vi "Dashboard Main.vi"() -> ()   [LabVIEW 2018]
uses:
  <vilib>/Rock Robotics/WPI/Camera/WPI_CameraExposure Values.ctl
  <vilib>/Rock Robotics/WPI/Camera/WPI_CameraWhite Balance Values.ctl
  <vilib>/Rock Robotics/WPI/Camera/WPI_CameraSettings Read MJPG.ctl
  <vilib>/Rock Robotics/WPI/Camera/WPI_CameraImageSize.ctl
  <vilib>/Utility/miscctls.llb/LVRowAndColumnTypeDef.ctl
  <vilib>/event_ctls.llb/eventvkey.ctl
  <vilib>/Rock Robotics/Network Tables/NT Read Numeric Array.vi
  <vilib>/Rock Robotics/WPI/Dashboard/WPI_DashboardLogging Global.vi
  <vilib>/Rock Robotics/Network Tables/NT Write Boolean.vi
  Vision Things/Dashboard globals.vi
  <vilib>/Utility/inputDevices.llb/keyboardAcquire.vi
  <vilib>/vision/NI_Vision_Development_Module.lvlib
  <vilib>/Rock Robotics/Network Tables/NT Write Variant.vi
panel:
  in  "Camera Settings Right":T1={"Frame Rate"=30, "Compression"=30, "Size"=1, "DB Camera Config"=FALSE} {"Frame Rate" scale=1.0..30.0; "Compression" scale=100.0..-1.0; "Size" items=["640x480", "320x240", "160x120"]}
  in  "Camera Name Right":string(combo)="No Camera Selection"
  out "Camera Perf":string
  in  "Camera Settings":T1={"Frame Rate"=30, "Compression"=30, "Size"=1, "DB Camera Config"=FALSE} {"Frame Rate" scale=1.0..30.0; "Compression" scale=100.0..-1.0; "Size" items=["640x480", "320x240", "160x120"]}
  in  "TCP":refnum<k5>
  in  "Rec Mode":enum32{"Stop", "Record", "Playback"}(radio)
  out "Robot IP":string
  out "Image Message":string="Timeout in Camera Communications"
  in  "Dashboard Tab":T2(tab)
  in  "Desired Target":T3(radio)
  in  "Select Auto":string(combo)="Select Autonomous ..."
  out "NT Connection":bool
  out "MotorChart R":cluster{"Numeric":dbl, "Numeric":dbl}(graph)
  out "MotorChart L":cluster{"Numeric":dbl, "Numeric":dbl}(graph)
  out "MotorSliders R":cluster{"MotorSlide1":dbl, "MotorSlide2":dbl} {"MotorSlide2" scale=-1.0..1.0 scale format="%#_2e"; "MotorSlide1" scale=-1.0..1.0 scale format="%#_2e"}
  out "MotorSliders L":cluster{"MotorSlide1":dbl, "MotorSlide2":dbl} {"MotorSlide2" scale=-1.0..1.0 scale format="%#_2e"; "MotorSlide1" scale=-1.0..1.0 scale format="%#_2e"}
  out "Gyro":dbl(knob) scale=0.0..360.0
  out "JS1 Z":dbl(slide) scale=-1.0..1.0 scale format="%#_2e"
  out "JS1 Graph":cluster{"X":dbl, "Y":dbl}[](graph)
  out "JS1 Buttons":T4
  out "JS2 Z":dbl(slide) scale=-1.0..1.0 scale format="%#_2e"
  out "JS2 Graph":cluster{"X":dbl, "Y":dbl}[](graph)
  out "JS2 Buttons":T4
  out "Mode":T5(ring)=enum."Auto Disabled"
  out "Right Camera Perf":cluster{"Bandwidth (Mbps)":dbl, "FPS":dbl}
  in  "Auton Side":enum16{"Front", "Left", "Right"}(ring)
  in  "Side Code":enum16{"Right", "Left"}(ring)
  in  "Slot #":enum16{"3", "2", "1"}(ring)
  out "Auton String":string
  in  "Starting Postion":enum16{"2R", "2L", "1L", "1R", "1M"}(ring)
  out "Camera Image Right":T6(plugin-control)
  in  "DB/String 9":string
  in  "DB/String 8":string
  in  "DB/String 7":string
  in  "DB/String 6":string
  in  "DB/String 5":string
  in  "DB/String 4":string
  in  "DB/String 3":string
  in  "DB/String 2":string
  in  "DB/String 1":string
  in  "DB/String 0":string
  in  "DB/Slider 0":dbl(slide) scale=0.0..5.0
  in  "DB/Slider 1":dbl(slide) scale=0.0..5.0
  in  "DB/Slider 2":dbl(slide) scale=0.0..5.0
  in  "DB/Slider 3":dbl(slide) scale=0.0..5.0
  out "DB/LED 3":bool
  out "DB/LED 2":bool
  out "DB/LED 1":bool
  out "DB/LED 0":bool
  in  "DB/Button 3":bool
  in  "DB/Button 2":bool
  in  "DB/Button 1":bool
  in  "DB/Button 0":bool caption="New Name"
  in  "Test Slider":dbl(slide) scale=0.0..100.0 scale format="%#_3g"
  in  "On/Off":bool caption="Solenoid"
  in  "Test Name":u16(ring) items=["Select the test to run..."]
  in  "Test Tree":string(tree)
  in  "Motor":cluster{"Value":dbl, "Enable":bool} {"Value" scale=-1.0..1.0 scale format="%#_3g"}
  out "Progress":T7 {"Test Progress" scale=0.0..100.0}
  in  "Rev/Fwd":cluster{"Forward":bool, "Reverse":bool}
  in  "Test Ring":u16(ring) items=["Monochrome", "Color"]
  out "Cmd Status":string
  in  "Execute Command":bool
  in  "Command Params":string[][](table)
  in  "Command Selection":i32(listbox)
  in  "CheckList":i32(listbox)
  out "Tree":string(tree)
  out "Camera Image":T6(plugin-control)
  out "Background":bool
  in  "Camera Name":string(combo)="No Camera Selection"
  # "HW"
  # "HW"
  # "Joysticks"
  # "Drive Motors"
  # "Front"
  # "Right"
  # "Left"
  # "Back"
  # "This tab is a great place for autonomous settings and robot-specific values.\nPlace controls and indicators inside this tab and match name to\nDashboard Variables on robot. You can also delete this comment."
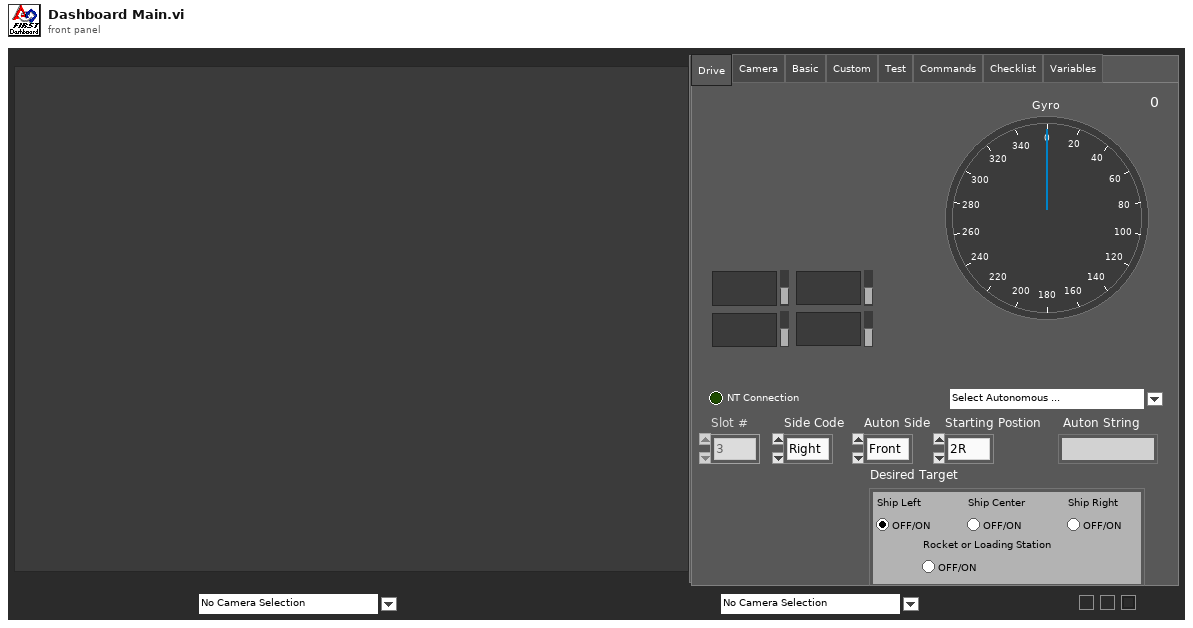
[diagram p1: front panel]
types:
  T1 = cluster{"Frame Rate":i32, "Compression":i32, "Size":u16, "DB Camera Config":bool}
  T2 = enum32{"Drive", "Camera", "Basic", "Custom", "Test", "Commands", "Checklist", "Variables"}
  T3 = enum32{"Ship Left", "Ship Center", "Ship Right", "Rocket or Loading Station"}
  T4 = cluster{bool, bool, bool, bool, bool, bool, bool, bool, bool, bool, bool, bool}
  T5 = enum8{"Tele-Op Disabled", "Tele-Op Enabled", "Auto Disabled", "Auto Enabled", "Test Disabled", "Test Enabled", "Disconnected", "No Code", "E-Stop"}
  T6 = typedef "IMAQ Image.ctl" = refnum<image>
  T7 = cluster{"Test Progress":u8, "Test Progress Text":string}
  T8 = cluster{"Save Path":path, "Interval (s)":dbl, "Keep":i32}
  T9 = typedef "Image Type" = u32
  T10 = cluster{"IDs":cluster{"RPC field ID":u16, "Unique ID":u16}, "String":string}
  T11 = enum8{"Enabled", "Disabled", "Disabled and Grayed Out"}
  T12 = enum16{"0", "1", "2", "3", "4", "5", "6", "7", "8", "9", "A", "B", "C", "D", "E", "F", "G", "H", "I", "J", "K", "L", "M", "N", "O", "P", "Q", "R", "S", "T", "U", "V", "W", "X", "Y", "Z", "F1", "F2", "F3", "F4", "F5", "F6", "F7", "F8", "F9", "F10", "F11", "F12", "F13", "F14", "F15", "ADD", "BACK", "BACKSLASH", "CAPITAL", "COMMA", "DECIMAL", "DELETE", "DIVIDE", "DOWN", "END", "EQUALS", "ESCAPE", "GRAVE (`)", "HOME", "INSERT", "LBRACKET", "LCONTROL", "LEFT", "L ALT", "LSHIFT", "LWIN", "MINUS", "MULTIPLY", "NEXT", "NUMLOCK", "NUMPAD_0", "NUMPAD_1", "NUMPAD_2", "NUMPAD_3", "NUMPAD_4", "NUMPAD_5", "NUMPAD_6", "NUMPAD_7", "NUMPAD_8", "NUMPAD_9", "PAUSE", "PERIOD", "PRIOR (PG UP)", "RBRACKET", "RCONTROL", "RETURN", "RIGHT", "R ALT", "RSHIFT", "RWIN", "SCROLL", "SEMICOLON", "SLASH", "SPACE", "SUBTRACT", "TAB", "UP", "ENTER (num pad)", "' (quote)"}[]
  T13 = enum16{"0", "1", "2", "3", "4", "5", "6", "7", "8", "9", "A", "B", "C", "D", "E", "F", "G", "H", "I", "J", "K", "L", "M", "N", "O", "P", "Q", "R", "S", "T", "U", "V", "W", "X", "Y", "Z", "F1", "F2", "F3", "F4", "F5", "F6", "F7", "F8", "F9", "F10", "F11", "F12", "F13", "F14", "F15", "ADD", "BACK", "BACKSLASH", "CAPITAL", "COMMA", "DECIMAL", "DELETE", "DIVIDE", "DOWN", "END", "EQUALS", "ESCAPE", "GRAVE (`)", "HOME", "INSERT", "LBRACKET", "LCONTROL", "LEFT", "L ALT", "LSHIFT", "LWIN", "MINUS", "MULTIPLY", "NEXT", "NUMLOCK", "NUMPAD_0", "NUMPAD_1", "NUMPAD_2", "NUMPAD_3", "NUMPAD_4", "NUMPAD_5", "NUMPAD_6", "NUMPAD_7", "NUMPAD_8", "NUMPAD_9", "PAUSE", "PERIOD", "PRIOR (PG UP)", "RBRACKET", "RCONTROL", "RETURN", "RIGHT", "R ALT", "RSHIFT", "RWIN", "SCROLL", "SEMICOLON", "SLASH", "SPACE", "SUBTRACT", "TAB", "UP", "ENTER (num pad)", "' (quote)"}
  T14 = typedef "WPI_CameraExposure Values.ctl" = enum16{"Auto", "Flicker-free 50 Hz", "Flicker-free 60 Hz", "Hold current", "Custom"}
  T15 = typedef "WPI_CameraWhite Balance Values.ctl" = enum16{"Auto", "Fixed indoor", "Fixed outdoor 1", "Fixed outdoor 2", "Fixed fluorescent 1", "Fixed fluorescent 2", "Hold current", "Custom"}
  T16 = cluster{"Exposure":T14, "Exposure (%)":dbl, "Brightness":i32, "White Balance":T15, "Color Temp (K)":dbl}
  T17 = typedef "WPI_CameraSettings Read MJPG.ctl" = cluster{"fps":i32, "compression":i32, "Image Size":T18, "Config Shown":bool}
  T18 = typedef "WPI_CameraImageSize.ctl" = enum16{"640x480", "320x240", "160x120", "Custom"}
  T19 = cluster{"Global Rectangle":i32[], "Contours":cluster{"Contour Type":u32, "ROI Type":u32, "Points":i32[]}[]}
  T20 = cluster{"Camera Name":string, string, "Saved DB Images Info":cluster{"Save Path":path, "Interval (s)":dbl, "Keep":i32}}
  T21 = cluster{"Corners":cluster{"X":sgl, "Y":sgl}[], "Orientation (degrees)":dbl, "Width":dbl, "Height":dbl, "Score":dbl}[]
  T22 = cluster{"Camera Name Right":string, string, "Saved DB Images Info":cluster{"Save Path":path, "Interval (s)":dbl, "Keep":i32}}
  T23 = cluster{"Camera Image":refnum<vi>, "Dashboard Tab":refnum<vi>, "Background":refnum<vi>, "Rec Mode":refnum<vi>, "Test Slider":refnum<vi>, "On/Off ":refnum<vi>, "Test Ring":refnum<vi>, "Rev/Fwd":refnum<vi>, "Test Name":refnum<vi>, "Motor":refnum<vi>, "Progress":refnum<vi>, "CheckList":refnum<vi>, "Tree":refnum<vi>, "Test Tree":refnum<vi>, "Command Params":refnum<vi>, "Command Selection":refnum<vi>, "Execute Command":refnum<vi>, "Cmd Status":refnum<vi>, "Camera Settings":refnum<vi>, "Camera Name":refnum<vi>, "Camera Perf":refnum<vi>, "Camera Settings Right":refnum<vi>, "Camera Name Right":refnum<vi>, "Camera Image Right":refnum<vi>}
  T24 = cluster{"Error Strings":string, "Disable Counts":cluster{u16, u16}, "Rail Faults":cluster{u16, u16, u16}, "Robot IP":string, "DB Mode":u8, "Event Info":cluster{"Name":string, "Type":u8, "Number":u16, "Replay":u8}}
  T25 = cluster{"Storage":cluster{"Disk Free":u64, "RAM Block":u32, "RAM free":u32}, "CPU Utilization":cluster{"CPU % ISR":sgl, "CPU % Time Crit":sgl, "CPU % Timed Str":sgl, "CPU % High":sgl, "CPU % Above":sgl, "CPU % Normal":sgl, "CPU % Low":sgl}, "CAN":cluster{"% Bus Utilization":sgl, "Bus Off Cnt":u32, "TX_FIFO Full Cnt":u32, "Receive Error Cnt":u8, "Transmit Error Cnt":u8}, "HID":cluster{"HID Outputs":u32, "Rumble Low":u16, "Rumble High":u16}[]}
  T26 = cluster{"Status bits":cluster{"Test Mode":bool, "Autonomous":bool, "Enabled":bool, "Code Start":bool, "Brownout":bool, "Reserved 2":bool, "Reserved 3":bool, "E-Stop":bool}, "Code Trace":cluster{"Disabled":bool, "TeleOp":bool, "Auto":bool, "Test":bool}, "Controller Type":enum16{"unknown", "cRIO", "roboRio"}, "Code?":enum16{"unknown", "noCode", "code"}, "Battery V":dbl}
  T27 = cluster{"Control Bits":cluster{"TestMode":bool, "Autonomous":bool, "Enabled":bool, "FMS Present":bool, bool, bool, bool, "E-Stop":bool}, "Team Station ":u8, "Countdown":sgl, "Joystick Values":cluster{"Axes":dbl[], "Buttons":bool[], "POVs":i16[]}[]}
  T28 = cluster{"Axes":dbl[], "Buttons":bool[], "POVs":i16[]}[]
  T29 = cluster{"Increase in Left":dbl, "Increase in Right":dbl}[]
  T30 = cluster{"Axes":dbl[], "Buttons":bool[], "POVs":i16[]}
  T31 = cluster{"Buttons[0]":bool, "Buttons[1]":bool, "Buttons[2]":bool, "Buttons[3]":bool, "Buttons[4]":bool, "Buttons[5]":bool, "Buttons[6]":bool, "Buttons[7]":bool, "Buttons[8]":bool, "Buttons[9]":bool, "Buttons[10]":bool, "Buttons[11]":bool}
  T32 = cluster{"Operation":enum16{"Update", "Clear"}, "Color Box":u32}[]
  T33 = typedef "eventvkey.ctl" = enum16{"ASCII", "Enter", "Return", "Shift", "Ctrl", "Alt", "Cmd", "Opt", "Caps", "NumLock", "Clear", "Break", "Up", "Down", "Left", "Right", "Insert", "Delete", "Home", "End", "PageUp", "PageDown", "Escape", "Help", "Pause", "ScrollLock", "F1", "F2", "F3", "F4", "F5", "F6", "F7", "F8", "F9", "F10", "F11", "F12", "F13", "F14", "F15", "F16", "F17", "F18", "F19", "F20", "F21", "F22", "F23", "F24", "Play", "VolumeUp", "VolumeDown", "Mute", "Two Byte Char"}
  T34 = cluster{"Image Size":bool, "Image Type":bool, "Pixel Value":bool, "ROI Information":bool, "Zoom Factor":bool}
  T35 = cluster{"Operation":enum16{"Update", "Clear"}, "Color Box":u32}
  T36 = typedef "LVRowAndColumnTypeDef.ctl" = cluster{"Row":i32, "Column":i32}
  T37 = cluster{"Shift":bool, "Ctrl":bool, "Alt":bool, "Cmd":bool, "Opt":bool}
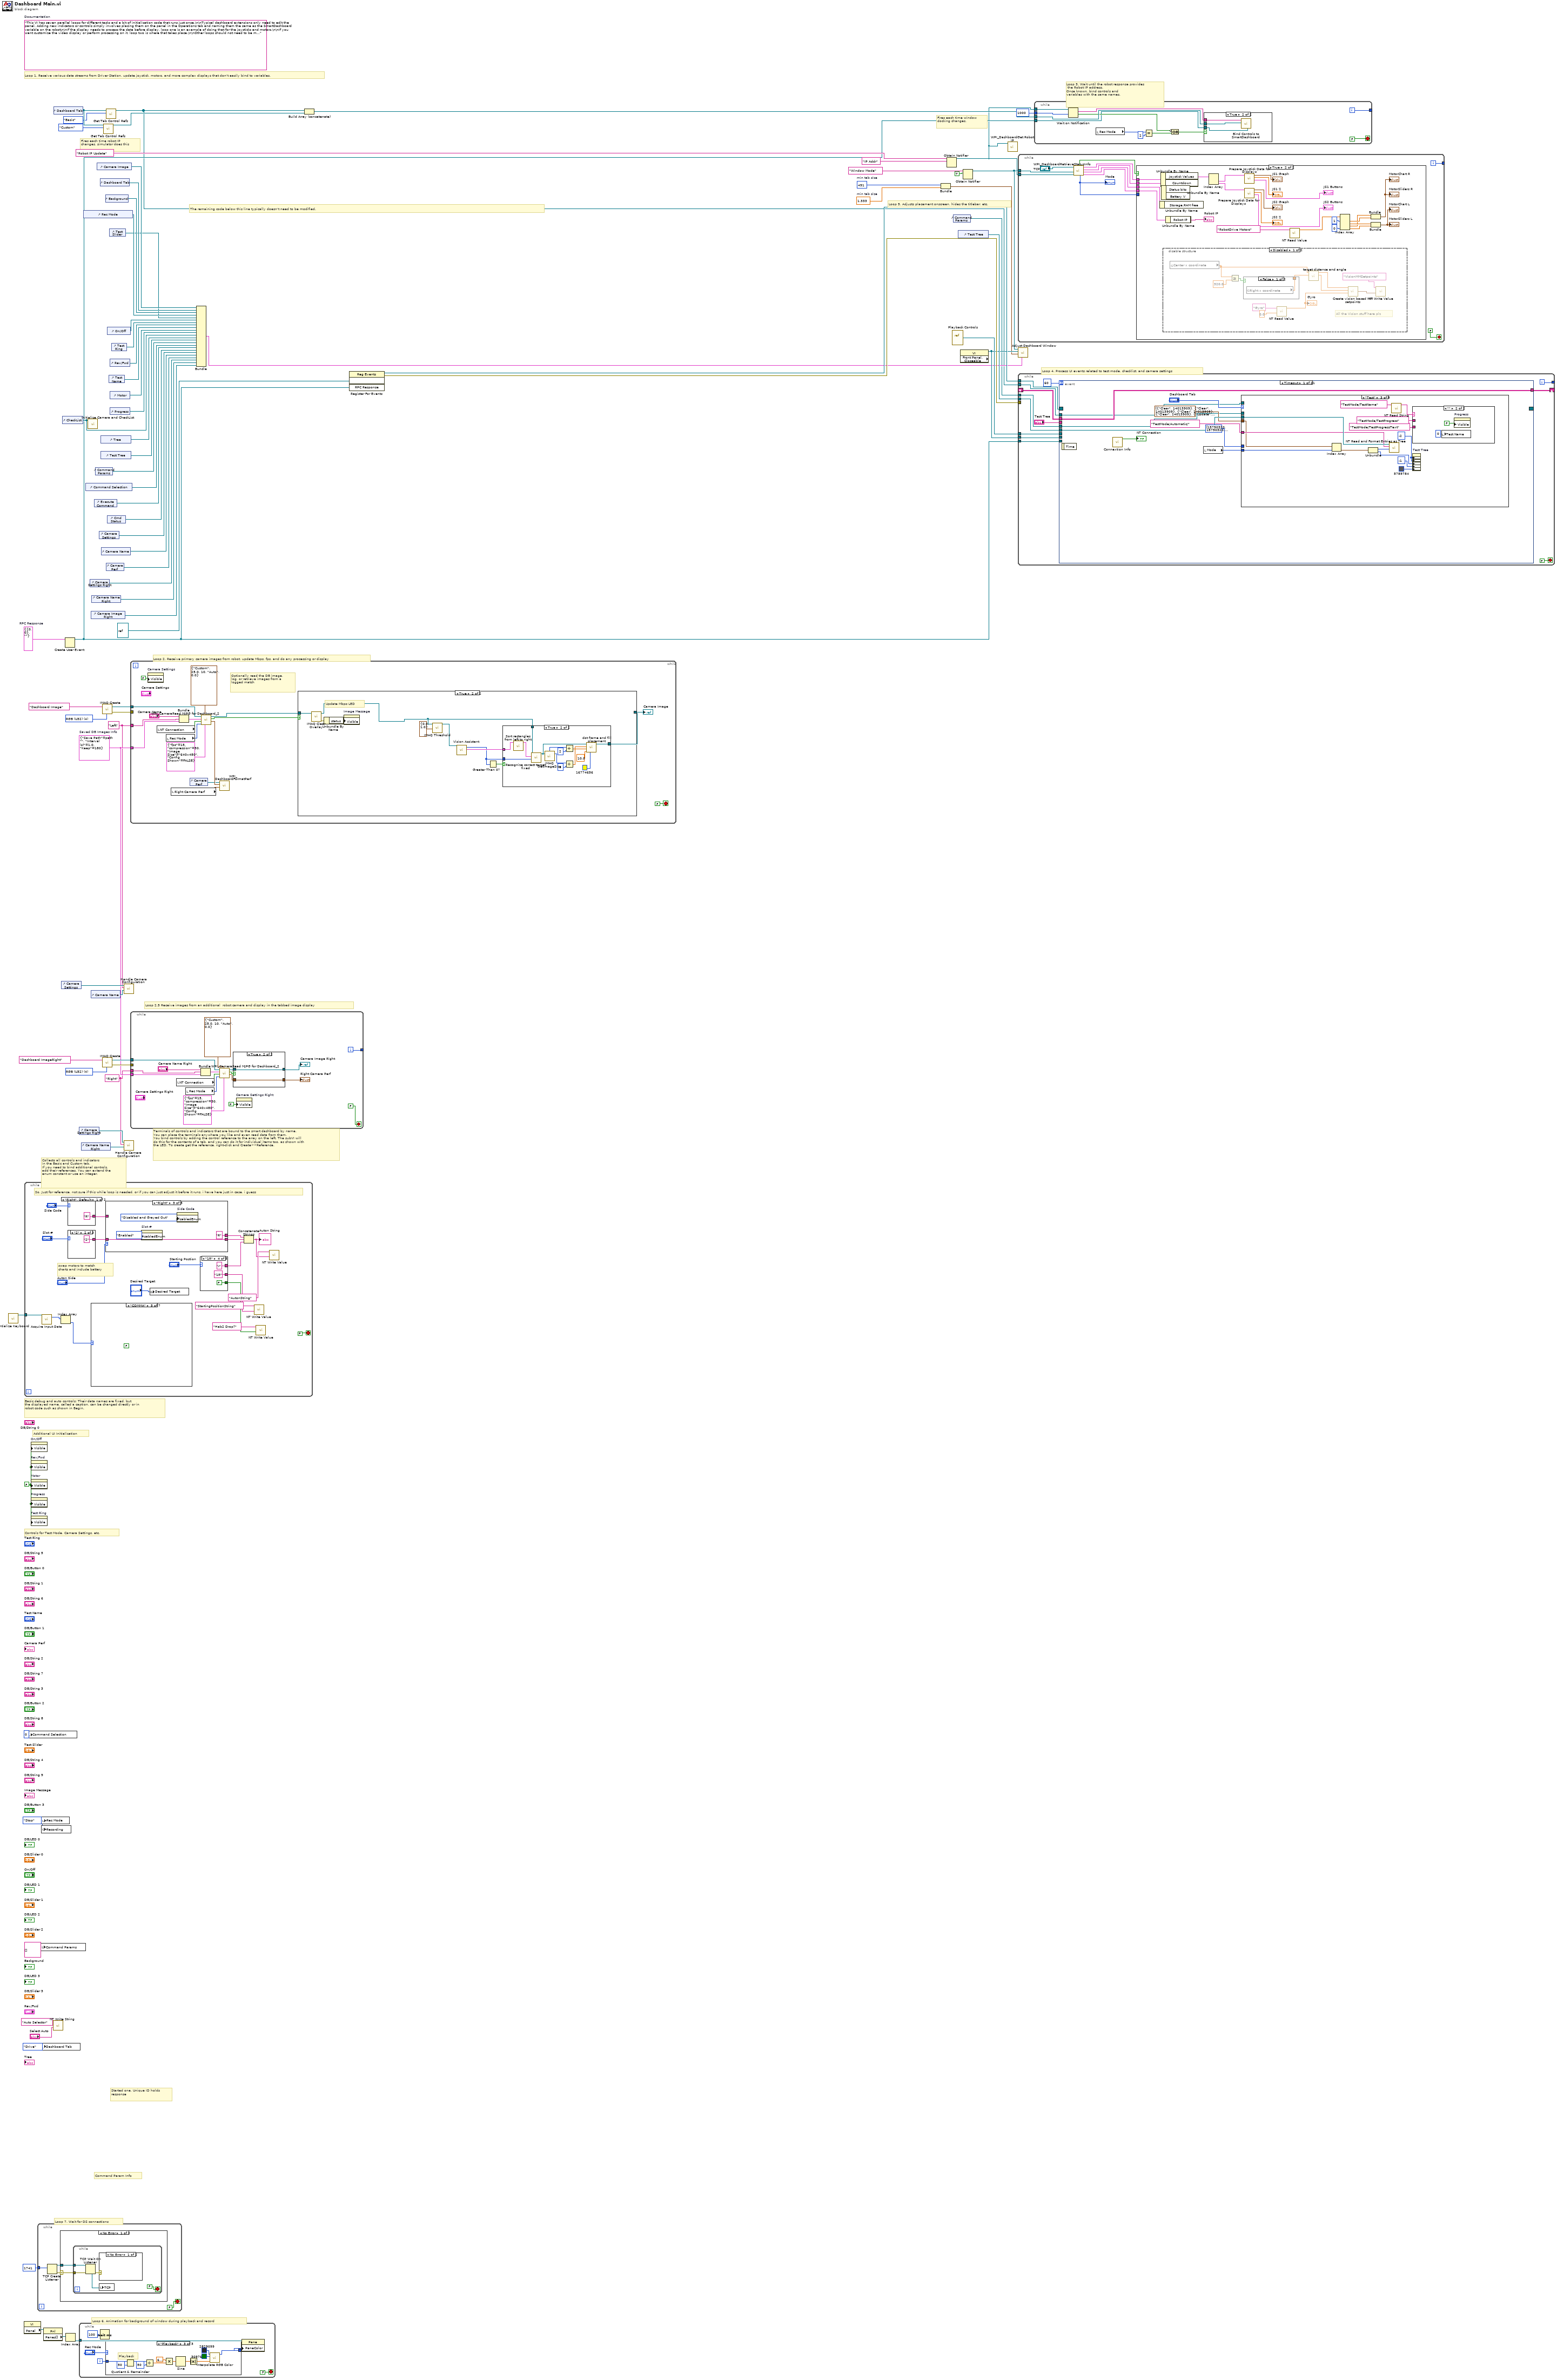
[diagram p0: block diagram]
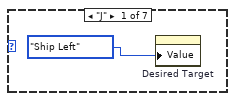
[diagram p2: hidden frame]
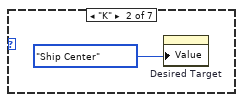
[diagram p3: hidden frame]
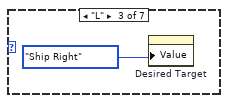
[diagram p4: hidden frame]
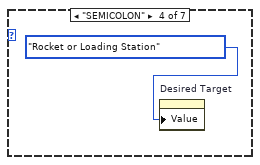
[diagram p5: hidden frame]
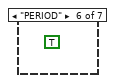
[diagram p6: hidden frame]
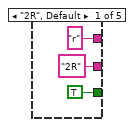
[diagram p8: hidden frame]
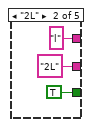
[diagram p9: hidden frame]
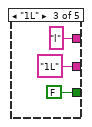
[diagram p10: hidden frame]
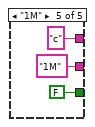
[diagram p11: hidden frame]
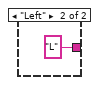
[diagram p12: hidden frame]
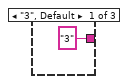
[diagram p13: hidden frame]
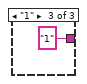
[diagram p14: hidden frame]
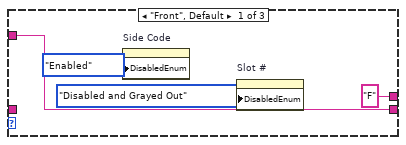
[diagram p15: hidden frame]
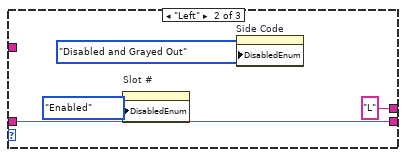
[diagram p16: hidden frame]
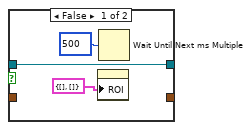
[diagram p17: hidden frame]
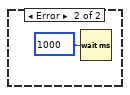
[diagram p18: hidden frame]
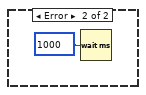
[diagram p19: hidden frame]
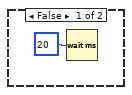
[diagram p20: hidden frame]
diagram:
  w5 = T8 {"Save Path"=path "", "Interval (s)"=1.0, "Keep"=180}  # Saved DB Images Info
  w4 = "Right"
  w3 = "Left"
  w15 = T9 4 items=["Grayscale (U8)", "Grayscale (I16)", "Grayscale (SGL)", "Complex (CSG)", "RGB (U32)", "HSL (U32)", "RGB (U64)"] ("Image Type")
  w31 = T10 {"IDs"={"RPC field ID"=0, "Unique ID"=0}, "String"=""}  # RPC Response
  w53 = 491  # min tab size
  w52 = 1.333  # min tab size
  w60 = enum32{"Stop", "Record", "Playback"}."Stop" ("Rec Mode")
  w37 = FALSE ("Visible")
  (unwired) "This VI has seven parallel loops for different tasks and a bit of initialization code that runs just once.\n\nTypical dashboard extensions only need to edit the panel. Adding new indicators or controls simply involves placing them on the panel in the Operations tab and naming them the same as the SmartDashboard variable on the robot\n\nIf the display needs to process the data before display, loop one is an example of doing that for the joysticks and motors.\n\nIf you want customize the video display or perform processing on it, loop two is where that takes place.\n\nOther loops should not need to be modified. They are pretty standard, and document the task they perform."  # Documentation
  w77 = T9 4 items=["Grayscale (U8)", "Grayscale (I16)", "Grayscale (SGL)", "Complex (CSG)", "RGB (U32)", "HSL (U32)", "RGB (U64)"] ("Image Type")
  # "Collects all controls and indicators\nin the Basic and Custom tab.\nIf you need to bind additional controls,\nadd their references. You can extend the\nenum constant or use an integer."
  # "Terminals of controls and indicators that are bound to the smart dashboard by name.\nYou can place the terminals anywhere you like and even read data from them.\nYou bind controls by adding the control reference to the array on the left. The subVI will\ndo this for the contents of a tab, and you can do it for individual items too, as shown with\nthe LED. To create get the reference, right-click and Create>>Reference."
  # "Loop 2.5 Receive images from an additional  robot camera and display in the tabbed image display"
  # "Command Param Info"
  # "Started one, Unique ID holds\nresponse"
  # "Loop 7. Wait for DS connections"
  # "Basic debug and auto controls: Their data names are fixed, but\nthe displayed name, called a caption, can be changed directly or in\nrobot code such as shown in Begin."
  # "Controls for Test Mode, Camera Settings, etc."
  # "Additional UI Initialization"
  # "Loop 6. Animation for background of window during playback and record"
  # "Fires each time robot IP\nchanges, simulator does this"
  # "Fires each time window\ndocking changes."
  # "The remaining code below this line typically doesn't need to be modified."
  # "Loop 4. Process UI events related to test mode, checklist, and camera settings"
  # "Loop 3. Wait until the robot response provides\n the Robot IP address.\nOnce known, bind controls and\nvariables with the same names."
  # "Loop 5. Adjusts placement onscreen, hides the titlebar, etc."
  # "Loop 1. Receive various data streams from Driver Station, update joystick, motors, and more complex displays that don't easily bind to variables."
  # "Loop 2. Receive primary camera images from robot, update Mbps, fps, and do any processing or display"
  n1 = call <vilib>:"Intialize Keyboard.vi"() -> ("device ID"=w2:refnum<k1>)  [unwired: 10 in, 1 out]
  n2 = property class="VI"() -> ("Panel"=w67:refnum<vi>)  [unwired: 2 in, 2 out]
  n3 = while {
    tunnel: w2 -> [w81]
    stop <- FALSE stop-if-true
    # "So, Just for reference, not sure if this while loop is needed, or if you can just adjust it before it runs, i have here just in case, i guess"
    # "swap motors to match\ncharts and include battery"
    n4 = call-poly <vilib>:"Acquire Input Data.vi"("device ID"=w81) -> ("keys pressed"=w80:T12)  [unwired: 16 in, 2 out]
    n5 = Index Array(array=w80) -> (element=w79:T13)  [unwired: 1 in]
    n6 = case shown="\"Right\", Default" "Side Code" {
      tunnel: ["R" "L"] -> w93
      frame "Right", Default {
      }
      frame "Left" {
      }
    }
    n7 = case shown="\"2\"" "Slot #" {
      tunnel: ["3" "2" "1"] -> w94
      frame "3", Default {
      }
      frame "2" {
      }
      frame "1" {
      }
    }
    n8 = case shown="\"COMMA\"" w79 {
      frame "J" {
        n9 = property on="Desired Target" class="RadioBtnsControl (strict)"("Value"=T3."Ship Left" ("Desired Target")) -> ()  [unwired: 2 in, 2 out]
      }
      frame "K" {
        n10 = property on="Desired Target" class="RadioBtnsControl (strict)"("Value"=T3."Ship Center" ("Desired Target")) -> ()  [unwired: 2 in, 2 out]
      }
      frame "L" {
        n11 = property on="Desired Target" class="RadioBtnsControl (strict)"("Value"=T3."Ship Right" ("Desired Target")) -> ()  [unwired: 2 in, 2 out]
      }
      frame "SEMICOLON" {
        n12 = property on="Desired Target" class="RadioBtnsControl (strict)"("Value"=T3."Rocket or Loading Station" ("Desired Target")) -> ()  [unwired: 2 in, 2 out]
      }
      frame "COMMA" {
        (unwired) FALSE ("Enable Vision Processing")
      }
      frame "PERIOD" {
        (unwired) TRUE ("Enable Vision Processing")
      }
      frame "0", Default {
      }
    }
    n13 = case shown="\"Right\"" "Auton Side" {
      tunnel: w94 -> [_ w126 w130]
      tunnel: w93 -> [w122 _ _]
      tunnel: [w122 w126 w130] -> w89
      tunnel: ["F" "L" "R"] -> w90
      frame "Front", Default {
        n14 = property on="Side Code" class="Enum (strict)"("DisabledEnum"=T11."Enabled" ("Disabled")) -> ()  [unwired: 2 in, 2 out]
        n15 = property on="Slot #" class="Enum (strict)"("DisabledEnum"=T11."Disabled and Grayed Out" ("Disabled")) -> ()  [unwired: 2 in, 2 out]
      }
      frame "Left" {
        n16 = property on="Slot #" class="Enum (strict)"("DisabledEnum"=T11."Enabled" ("Disabled")) -> ()  [unwired: 2 in, 2 out]
        n17 = property on="Side Code" class="Enum (strict)"("DisabledEnum"=T11."Disabled and Grayed Out" ("Disabled")) -> ()  [unwired: 2 in, 2 out]
      }
      frame "Right" {
        n18 = property on="Slot #" class="Enum (strict)"("DisabledEnum"=T11."Enabled" ("Disabled")) -> ()  [unwired: 2 in, 2 out]
        n19 = property on="Side Code" class="Enum (strict)"("DisabledEnum"=T11."Disabled and Grayed Out" ("Disabled")) -> ()  [unwired: 2 in, 2 out]
      }
    }
    n20 = global write "Dashboard globals.vi" "Desired Target"("Desired Target") -> ()
    n21 = case shown="\"1R\"" "Starting Postion" {
      tunnel: ["2R" "2L" "1L" "1R" "1M"] -> w86
      tunnel: [TRUE TRUE FALSE FALSE FALSE] -> w83
      tunnel: ["r" "l" "l" "r" "c"] -> w82
      frame "2R", Default {
      }
      frame "2L" {
      }
      frame "1L" {
      }
      frame "1R" {
      }
      frame "1M" {
      }
    }
    n22 = Concatenate Strings(w90, w89, w82) -> (w87:string)
    "Auton String" <- w87
    n23 = call-poly <vilib>:"NT Write Value.vi"("String"=w86, "Name"="StartingPositionString") -> ()  [unwired: 9 in, 1 out]
    n24 = call-poly <vilib>:"NT Write Value.vi"("Boolean"=w83, "Name"="Hab2 Drop?") -> ()  [unwired: 9 in, 1 out]
    n25 = call-poly <vilib>:"NT Write Value.vi"("String"=w87, "Name"="AutonString") -> ()  [unwired: 9 in, 1 out]
  }
  n26 = local write "Command Selection"(u16 0 ("milliseconds to wait")) -> ()
  n27 = property on="On/Off" class="Bool (strict)"("Visible"=w37) -> ()  [unwired: 2 in, 2 out]
  n28 = property on="Rev/Fwd" class="Clust (strict)"("Visible"=w37) -> ()  [unwired: 2 in, 2 out]
  n29 = property on="Motor" class="Clust (strict)"("Visible"=w37) -> ()  [unwired: 2 in, 2 out]
  n30 = property on="Progress" class="Clust (strict)"("Visible"=w37) -> ()  [unwired: 2 in, 2 out]
  n31 = property on="Test Ring" class="Ring (strict)"("Visible"=w37) -> ()  [unwired: 2 in, 2 out]
  n32 = while {
    tunnel: u16 1741 ("timeout ms (25000)") -> [w135]
    stop <- FALSE stop-if-true
    n33 = TCP Create Listener(10:w135) -> (0:w134:errorcluster, 3:w136:refnum<k5>)  [unwired: 4 in, 1 out]
    n34 = case shown="No Error" w134 {
      selector: w134 -> [w138 _]
      tunnel: w136 -> [w139 _]
      frame No Error {
        n35 = while {
          tunnel: w139 -> [w142]
          tunnel: w138 -> [w141]
          stop <- FALSE stop-if-true
          n36 = TCP Wait On Listener(8:w141, 11:w142) -> (0:w143:errorcluster, 4:w144:refnum<k5>)  [unwired: 2 in, 3 out]
          n37 = local write "TCP"(w144) -> ()
          n38 = case shown="No Error" w143 {
            frame No Error {
            }
            frame Error {
              n39 = Wait (ms)(milliseconds to wait=u32 1000) -> ()  [unwired: 1 out]
            }
          }
        }
      }
      frame Error {
        n40 = Wait (ms)(milliseconds to wait=u32 1000) -> ()  [unwired: 1 out]
      }
    }
  }
  n41 = local write "Command Params"(string[][] [] ("Command Params")) -> ()
  n42 = local write "Dashboard Tab"(T2."Drive" ("Dashboard Tab")) -> ()
  n43 = local write "Rec Mode"(w60) -> ()
  n44 = global write "WPI_DashboardLogging Global.vi" "Recording"(w60) -> ()
  n45 = property class="Pnl"(reference=w67) -> ("Panes[]"=w68:refnum<vi>[])  [unwired: 1 in, 2 out]
  n46 = call <vilib>:"NT Write String.vi"("String"="Select Auto", "Name"="Auto Selector") -> ()  [unwired: 9 in, 1 out]
  n47 = control-ref of="Dashboard Tab"() -> (w58:refnum<vi>)
  n48 = control-ref of="Camera Settings"() -> (w24:refnum<vi>)
  n49 = control-ref of="CheckList"() -> (w48:refnum<vi>)
  n50 = Create User Event(user event datatype=w31) -> (user event=w27:refnum<user-event>)  [unwired: 1 in, 1 out]
  n51 = Index Array(array=w68) -> (element=w66:refnum<vi>)  [unwired: 1 in]
  n52 = while {
    tunnel: w66 -> [w148]
    i -> [w151]
    stop <- FALSE stop-if-true
    n53 = Wait (ms)(milliseconds to wait=u32 100) -> ()  [unwired: 1 out]
    n54 = case shown="\"Playback\"" "Rec Mode" {
      tunnel: w151 -> [_ _ w166]
      tunnel: [u32 2829099 ("Base Color") u32 11141120 ("Target Color") w155] -> w147
      frame "Stop", Default {
        # "Reset the color, extra updates don't cost much"
      }
      frame "Record" {
      }
      frame "Playback" {
        # "Playback"
        n55 = Quotient & Remainder(x=w166, y=u32 50 ("milliseconds to wait")) -> (x-y*floor(x/y)=w162:u32)  [unwired: 1 out]
        n56 = Divide(x=w162, y=u32 50 ("milliseconds to wait")) -> (x/y=w159:dbl)
        n57 = Multiply(x=6.283185307179586, y=w159) -> (x*y=w164:dbl)
        n58 = Sine(x=w164) -> (sin(x)=w163:dbl)
        n59 = Absolute Value(x=w163) -> (abs(x)=w156:dbl)
        n60 = call "Interpolate RGB Color.vi"("Proportion"=w156, "Target Color"=u32 30976, "Base Color"=u32 2829099) -> ("Result Color"=w155:u32)  [unwired: 8 in]
      }
    }
    n61 = property class="Pane"(reference=w148, "PaneColor"=w147) -> ()  [unwired: 1 in, 2 out]
  }
  n62 = control-ref of="Camera Settings Right"() -> (w12:refnum<vi>)
  n63 = control-ref of="Camera Name Right"() -> (w11:refnum<vi>)
  n64 = control-ref of="Rec Mode"() -> (w43:refnum<vi>)
  n65 = control-ref of="Command Selection"() -> (w30:refnum<vi>)
  n66 = call "Initialize Camera and CheckList.vi"("ListBox in"=w48) -> ()  [unwired: 11 in]
  n67 = control-ref of="Camera Settings Right"() -> (w10:refnum<vi>)
  n68 = control-ref of="Camera Image Right"() -> (w8:refnum<vi>)
  n69 = control-ref of="Camera Name"() -> (w23:refnum<vi>)
  n70 = control-ref of="Camera Name Right"() -> (w9:refnum<vi>)
  n71 = control-ref of="Execute Command"() -> (w32:refnum<vi>)
  n72 = control-ref of="Command Params"() -> (w33:refnum<vi>)
  n73 = control-ref of="Camera Image"() -> (w55:refnum<vi>)
  n74 = control-ref of="Camera Settings"() -> (w22:refnum<vi>)
  n75 = control-ref of="Dashboard Tab"() -> (w54:refnum<vi>)
  n76 = control-ref of="Tree"() -> (w47:refnum<vi>)
  n77 = control-ref of="Test Tree"() -> (w46:refnum<vi>)
  n78 = control-ref of="Camera Name"() -> (w21:refnum<vi>)
  n79 = call "IMAQ Create"("Image Name"="Dashboard Image", "Image Type"=w77) -> ("New Image"=w75:T6, "error out"=w74:errorcluster)  [unwired: 2 in, 1 out]
  n80 = call "IMAQ Create"("Image Name"="Dashboard ImageRight", "Image Type"=w15) -> ("New Image"=w14:T6, "error out"=w13:errorcluster)  [unwired: 2 in, 1 out]
  n81 = call <vilib>:"Get Tab Control Refs.vi"("Page Index"=T2."Custom" ("Dashboard Tab"), "TabControl in"=w58) -> ("ControlsOnPage"=w57:refnum<vi>[])  [unwired: 9 in]
  n82 = control-ref of="Background"() -> (w50:refnum<vi>)
  n83 = call <vilib>:"Get Tab Control Refs.vi"("Page Index"=T2."Basic" ("Dashboard Tab"), "TabControl in"=w58) -> ("ControlsOnPage"=w19:refnum<vi>[])  [unwired: 9 in]
  n84 = control-ref of="Camera Perf"() -> (w20:refnum<vi>)
  n85 = control-ref of="On/Off"() -> (w41:refnum<vi>)
  n86 = control-ref of="Cmd Status"() -> (w26:refnum<vi>)
  n87 = control-ref of="Test Name"() -> (w45:refnum<vi>)
  n88 = control-ref of="Test Slider"() -> (w42:refnum<vi>)
  n89 = control-ref of="Rev/Fwd"() -> (w39:refnum<vi>)
  n90 = control-ref of="Motor"() -> (w44:refnum<vi>)
  n91 = control-ref of="Progress"() -> (w38:refnum<vi>)
  n92 = control-ref of="Test Ring"() -> (w40:refnum<vi>)
  n93 = call "Handle Camera Configuration.vi"("CameraNameRef"=w23, "Display Name"=w3, "ClusterRef"=w24) -> ()  [unwired: 9 in]
  n94 = call "Handle Camera Configuration.vi"("CameraNameRef"=w11, "Display Name"=w4, "ClusterRef"=w12) -> ()  [unwired: 9 in]
  n95 = while {
    tunnel: w75 -> [w182]
    tunnel: w74 -> [_]
    tunnel: w5 -> [w176]
    tunnel: w3 -> [w173]
    stop <- FALSE stop-if-true
    # "Optionally read the DB image,\nlog, or retrieve images from a\nlogged match"
    n96 = property on="Camera Settings" class="Clust (strict)"("Visible"=FALSE) -> ()  [unwired: 2 in, 2 out]
    n97 = local read "NT Connection"() -> (w177:bool)
    n98 = local read "Rec Mode"() -> (w179:enum32{"Stop", "Record", "Playback"})
    n99 = local read "Right Camera Perf"() -> (w171:cluster{"Bandwidth (Mbps)":dbl, "FPS":dbl})
    n100 = Bundle("Camera Name"="Camera Name", w173, "Saved DB Images Info"=w176) -> (w175:T20)  [unwired: 1 in]
    n101 = control-ref of="Camera Perf"() -> (w170:refnum<vi>)
    n102 = call <vilib>:"WPI_CameraRead MJPG for Dashboard_2.vi"("Camera Settings"=T17 {"fps"=15, "compression"=30, "Image Size"=enum."640x480", "Config Shown"=FALSE}, "Camera Settings 2"=T16 {"Exposure"=enum."Custom", "Exposure (%)"=25.0, "Brightness"=10, "White Balance"=enum."Auto", "Color Temp (K)"=0.0}, "Rec Mode"=w179, "NT Connection"=w177, "Capture Info"=w175, "Image in"=w182) -> ("perf info"=w172:cluster{"Bandwidth (Mbps)":dbl, "fps":dbl}, "Active"=w180:bool, "Image\\ out"=w181:T6)  [unwired: 3 in]
    n103 = call <vilib>:"WPI_DashboardFormatPerf.vi"("Right Camera Perf"=w171, "Performance"=w172, "String in"=w170) -> ()  [unwired: 9 in]
    n104 = case shown="True" w180 {
      tunnel: w181 -> [w185 w194]
      tunnel: [w185 w192] -> w178
      frame False {
        # "Sleep for 500ms"
        n105 = Wait Until Next ms Multiple(millisecond multiple=u32 500) -> ()  [unwired: 1 out]
        n106 = property on="Camera Image" class="ImageControl"("ROI"=T19 {"Global Rectangle"=[], "Contours"=[]}) -> ()  [unwired: 2 in, 2 out]
      }
      frame True {
        # "Update Mbps LED"
        n107 = call "IMAQ Clear Overlay"("Image"=w194) -> ("error out"=w195:errorcluster, "Image Out"=w193:T6)  [unwired: 2 in, 7 out]
        n108 = Unbundle By Name(w195) -> ("status"=w196:bool)
        n109 = property on="Image Message" class="Str"("Visible"=w196) -> ()  [unwired: 2 in, 2 out]
        n110 = call "IMAQ Threshold"("Range"=cluster{"Lower value":sgl, "Upper value":sgl} {"Lower value"=0.0, "Upper value"=1.0}, "Image Src"=w193) -> ("Image Dst Out"=w190:T6)  [unwired: 8 in, 1 out]
        n111 = call "Vision Assistant"("Image In"=w190) -> ("Number of Matches (Shape Detection 1)"=w187:i32, "Rectangles Calibrated (Shape Detection 1)"=w188:T21)  [unwired: 23 in, 2 out]
        n112 = Greater Than 0?(x=w187) -> (x > 0?=w189:bool)
        n113 = case shown="True" w189 {
          tunnel: w193 -> [w197 w211]
          tunnel: w188 -> [_ w210]
          tunnel: w187 -> [_ w209]
          tunnel: [w197 w199] -> w192
          frame False {
          }
          frame True {
            n114 = call "Sort rectangles from left to right.vi"("Rectangles (Calibrated) IN"=w210) -> ("Rectangles (Calibrated) OUT"=w208:T21)  [unwired: 10 in]
            n115 = call "Recognize correct target fixed.vi"("# rectangles"=w209, "Rectangles (Calibrated)"=w208, "Image"=w211) -> ("Image Out"=w207:T6)  [unwired: 8 in]
            n116 = call "IMAQ GetImageSize"("Image"=w207) -> ("Y Resolution"=w205:i32, "X Resolution"=w206:i32)  [unwired: 3 in, 1 out]
            n117 = Divide(x=w206, y=2) -> (x/y=w203:dbl)
            n118 = Divide(x=w205, y=2) -> (x/y=w204:dbl)
            n119 = call "dot frame and fill placement.vi"("Color"=u32 16774656, "size"=sgl 10.0, "y coordinate"=w204, "x coordinate"=w203, "Image"=w207) -> ("Image Out"=w199:T6)  [unwired: 6 in]
          }
        }
      }
    }
    "Camera Image" <- w178
  }
  n120 = while {
    tunnel: w14 -> [w228]
    tunnel: w13 -> [_]
    tunnel: [w224] -> _
    tunnel: w5 -> [w220]
    tunnel: w4 -> [w217]
    i -> [w224]
    stop <- FALSE stop-if-true
    n121 = local read "NT Connection"() -> (w221:bool)
    n122 = local read "Rec Mode"() -> (w227:enum32{"Stop", "Record", "Playback"})
    n123 = Bundle("Camera Name Right"="Camera Name Right", w217, "Saved DB Images Info"=w220) -> (w219:T22)  [unwired: 1 in]
    n124 = call <vilib>:"WPI_CameraRead MJPG for Dashboard_2.vi"("Camera Settings"=T17 {"fps"=15, "compression"=30, "Image Size"=enum."640x480", "Config Shown"=FALSE}, "Camera Settings 2"=T16 {"Exposure"=enum."Custom", "Exposure (%)"=25.0, "Brightness"=10, "White Balance"=enum."Auto", "Color Temp (K)"=0.0}, "Rec Mode"=w227, "NT Connection"=w221, "Capture Info"=w219, "Image in"=w228) -> ("perf info"=w215:cluster{"Bandwidth (Mbps)":dbl, "fps":dbl}, "Active"=w223:bool, "Image\\ out"=w226:T6)  [unwired: 3 in]
    n125 = case shown="True" w223 {
      tunnel: w226 -> [w230 w233]
      tunnel: [w230 w233] -> w222
      tunnel: [_ w232] -> w216
      tunnel: w215 -> [_ w232]
      frame False {
        n126 = property on="Camera Image Right" class="ImageControl"("ROI"=T19 {"Global Rectangle"=[], "Contours"=[]}) -> ()  [unwired: 2 in, 2 out]
        n127 = Wait Until Next ms Multiple(millisecond multiple=u32 500) -> ()  [unwired: 1 out]
      }
      frame True {
      }
    }
    "Camera Image Right" <- w222
    "Right Camera Perf" <- w216
    n128 = property on="Camera Settings Right" class="Clust (strict)"("Visible"=FALSE) -> ()  [unwired: 2 in, 2 out]
  }
  n129 = Bundle("Camera Image"=w55, "Dashboard Tab"=w54, "Background"=w50, "Rec Mode"=w43, "Test Slider"=w42, "On/Off"=w41, "Test Ring"=w40, "Rev/Fwd"=w39, "Test Name"=w45, "Motor"=w44, "Progress"=w38, "CheckList"=w48, "Tree"=w47, "Test Tree"=w46, "Command Params"=w33, "Command Selection"=w30, "Execute Command"=w32, "Cmd Status"=w26, "Camera Settings"=w22, "Camera Name"=w21, "Camera Perf"=w20, "Camera Settings Right"=w10, "Camera Name Right"=w9, "Camera Image Right"=w8) -> (w49:T23)  [unwired: 1 in]
  n130 = Build Array (concatenate)(w19, w57) -> (w56:refnum<vi>[])
  n131 = register-events(refnum<vi> refnum, w27) -> (reference out=w64:refnum<event-registration>, error out=w63:errorcluster)  [unwired: 2 in]
  n132 = Bundle("min tab size"=w53, "min tab size"=w52) -> (w51:cluster{"min tab size":i32, "min tab size":dbl})  [unwired: 1 in]
  n133 = Obtain Notifier(name (unnamed)="Robot IP Update", notification data type="IP Addr" ("name (unnamed)")) -> (notifier out=w1:refnum<notifier>)  [unwired: 2 in, 2 out]
  n134 = vi-ref "Playback Controls.vi"() -> (w65:refnum<vi>)
  n135 = control-ref of="Command Params"() -> (w25:refnum<vi>)
  n136 = control-ref of="Test Tree"() -> (w69:refnum<vi>)
  n137 = property class="VI" props=["Front Panel.Closeable"]() -> (reference out=w59:refnum<vi>)  [unwired: 2 in, 2 out]
  n138 = Obtain Notifier(name (unnamed)="Window Mode", notification data type=TRUE) -> (notifier out=w36:refnum<notifier>)  [unwired: 2 in, 2 out]
  n139 = call <vilib>:"WPI_DashboardGet Robot IP.vi"("Notifier in"=w1) -> ()  [unwired: 11 in]
  n140 = while {
    tunnel: [w243] -> _
    tunnel: w1 -> [w237]
    tunnel: w36 -> [w234]
    i -> [w243]
    stop <- FALSE stop-if-true
    n141 = call <vilib>:"WPI_DashboardRetrieveStatusInfo.vi"("Binding Refnum"=w237, "Window Mode Notifier"=w234, "TCP Cnx"="TCP") -> ("Power and Errors"=w238:T24, "Robot Metrics"=w241:T25, "Status Info"=w242:T26, "Control Info"=w239:T27, "Robot Mode"=w236:T5, "Process?"=w240:bool)  [unwired: 3 in]
    "Mode" <- w236
    n142 = case shown="True" w240 {
      tunnel: w242 -> [_ w269]
      tunnel: w241 -> [_ w268]
      tunnel: w239 -> [_ w267]
      tunnel: w238 -> [_ w266]
      tunnel: w236 -> [_ _]
      frame False {
        n143 = Wait (ms)(milliseconds to wait=u32 20) -> ()  [unwired: 1 out]
      }
      frame True {
        n144 = Unbundle By Name(w268) -> ()  [unwired: 1 out]
        n145 = Unbundle By Name(w267) -> ("Joystick Values"=w257:T28)  [unwired: 1 out]
        n146 = Unbundle By Name(w269) -> ()  [unwired: 2 out]
        n147 = disable-structure shown="Disabled" {
          frame Disabled {
            # "All the Vision stuff here plz"
            n148 = global read "Dashboard globals.vi" "Center x coordinate"() -> (w271:sgl)
            n149 = Greater Or Equal?(x=w271, y=sgl 320.0) -> (x >= y?=w273:bool)
            n150 = case shown="False" w273 {
              tunnel: [w281 w282] -> w270
              frame False {
                n151 = global read "Dashboard globals.vi" "Right x coordinate"() -> (w281:sgl)
              }
              frame True {
                n152 = global read "Dashboard globals.vi" "Left x coordinate"() -> (w282:sgl)
              }
            }
            n153 = call-poly <vilib>:"NT Read Value.vi"("Default Value"=0.0, "Name"="Gyro") -> ("Numeric"=w276:dbl)  [unwired: 8 in, 1 out]
            "Gyro" <- w276
            n154 = call "target distance and angle.vi"("x side"=w270, "x center"=w271) -> ("target angle in degrees"=w274:dbl, "distance from target in inches"=w275:dbl)  [unwired: 8 in]
            n155 = call "Create vision based MM setpoints.vi"("Gyro"=w276, "(phi) Vision's angle that the target is offcenter"=w274, "(I) Vision's distance to target"=w275) -> ("Vision-based MM Setpoints"=w279:T29)  [unwired: 1 in]
            n156 = call-poly <vilib>:"NT Write Value.vi"("Variant"=w279, "Name"="VisionMMSetpoints") -> ()  [unwired: 9 in, 1 out]
          }
          frame Enabled {
          }
        }
        n157 = Unbundle By Name(w266) -> ("Robot IP"=→"Robot IP":string)
        n158 = Index Array(array=w257) -> (element #1=w256:T30, element #2=w252:T30)  [unwired: 2 in]
        n159 = call "Prepare Joystick Data for Displays.vi"("Joystick Values"=w256) -> ("Buttons"=→"JS1 Buttons":T31, "Z Axis"=→"JS1 Z":dbl, "Cartesian Data"=→"JS1 Graph":cluster{"X axis":dbl, "X axis":dbl}[])  [unwired: 8 in]
        n160 = call "Prepare Joystick Data for Displays.vi"("Joystick Values"=w252) -> ("Buttons"=→"JS2 Buttons":T31, "Z Axis"=→"JS2 Z":dbl, "Cartesian Data"=→"JS2 Graph":cluster{"X axis":dbl, "X axis":dbl}[])  [unwired: 8 in]
        n161 = call-poly <vilib>:"NT Read Value.vi"("Name"="RobotDrive Motors") -> ("Numeric Array"=w247:dbl[])  [unwired: 9 in, 1 out]
        n162 = Index Array(array=w247, index #1=1, index #4=0) -> (element #1=w261:dbl, element #2=w262:dbl, element #3=w260:dbl, element #4=w265:dbl)  [unwired: 2 in]
        n163 = Bundle("Numeric"=w260, "Numeric"=w261) -> (→"MotorChart R" →"MotorSliders R":cluster{"Numeric":dbl, "Numeric":dbl})  [unwired: 1 in]
        n164 = Bundle("Numeric"=w262, "Numeric"=w265) -> (→"MotorChart L" →"MotorSliders L":cluster{"Numeric":dbl, "Numeric":dbl})  [unwired: 1 in]
      }
    }
  }
  n165 = call "Adjust Dashboard Window.vi"("Sizing Refnums"=w49, "Size Constraints"=w51, "VI"=w59, "WIn Mode"=w36) -> ()  [unwired: 8 in]
  n166 = while {
    tunnel: [w292] -> _
    tunnel: w69 -> [w291]
    tunnel: w65 -> [w290]
    tunnel: w64 -> [w289]
    tunnel: w63 -> [_]
    tunnel: w59 -> [w288]
    tunnel: w27 -> [w287]
    tunnel: w25 -> [w286]
    shift-right: [w285] -> _
    shift-left: _ -> [w284]
    tunnel: w19 -> [w283]
    i -> [w292]
    stop <- FALSE stop-if-true
    n167 = event shown="[0] Timeout" {
      selector: w289 -> [_ _ _ _ _ _ _ _ _ _ _ _ _ _ _ _ _ _ _ _ _]
      dyn-events: [_ _ _ _ _ _ _ _ _ _ _ _ _ _ _ _ w552 _ _ _ _] -> _
      timeout: u32 60 ("milliseconds to wait") -> [_ _ _ _ _ _ _ _ _ _ _ _ _ _ _ _ _ _ _ _ _]
      tunnel: w291 -> [w304 _ _ _ _ _ _ _ _ _ _ _ _ _ _ _ _ _ _ _ _]
      tunnel: "Test Tree" -> [_ _ _ _ _ _ _ _ _ _ _ w519 w527 w529 w533 w541 _ _ _ _ _]
      tunnel: w290 -> [_ _ _ _ _ _ _ _ _ _ _ _ _ _ _ _ w554 _ w572 _ _]
      tunnel: w288 -> [_ _ _ _ _ _ _ _ _ _ _ _ _ _ _ _ w550 _ _ _ _]
      tunnel: w287 -> [_ _ _ _ _ _ _ _ _ _ _ _ _ _ _ _ w548 _ _ _ _]
      tunnel: w286 -> [w299 _ _ _ _ _ w470 _ _ _ _ _ _ _ _ _ _ _ _ _ _]
      tunnel: [w298 w347 w449 w454 w463 w467 w468 w477 w487 w494 w506 w518 w525 w528 w532 w540 w547 w567 w569 w573 w586] -> w285
      tunnel: w284 -> [w298 w347 w449 w454 w463 w467 w468 _ _ w494 w506 w518 w525 w528 w532 w540 w547 w567 w569 w573 w586]
      tunnel: w283 -> [w296 _ _ _ _ _ _ _ _ _ _ _ _ _ _ _ _ _ _ _ _]
      event Timeout {
        n168 = event-data() -> ()  [unwired: 1 in, 1 out]
        n169 = call <vilib>:"Connextion Info.vi"() -> ("Connected"=→"NT Connection":bool)  [unwired: 10 in, 1 out]
        n170 = local read "Mode"() -> (w301:T5)
        n171 = case shown="\"Test\"" "Dashboard Tab" {
          tunnel: w304 -> [_ _ w320 _ _]
          tunnel: "TestMode/Automatic/" ("Name Pattern") -> [_ _ w319 _ _]
          tunnel: T32 [{"Operation"=enum."Clear", "Color Box"=14013909}, {"Operation"=enum."Clear", "Color Box"=14013909}, {"Operation"=enum."Clear", "Color Box"=14013909}, {"Operation"=enum."Clear", "Color Box"=14013909}, {"Operation"=enum."Update", "Color Box"=14013909}, {"Operation"=enum."Update", "Color Box"=16777215}, {"Operation"=enum."Clear", "Color Box"=14013909}, {"Operation"=enum."Clear", "Color Box"=14013909}, {"Operation"=enum."Clear", "Color Box"=14013909}] -> [_ _ w312 _ w340]
          tunnel: w301 -> [_ _ w311 _ w339]
          tunnel: u32[] [15790320, 15790320, 15790320, 15790320, 16777215, 16777215, 15790320, 15790320, 15790320] -> [_ _ _ _ w345]
          tunnel: w299 -> [_ _ _ _ w333]
          tunnel: w296 -> [_ w306 _ _ _]
          frame "Custom", Default {
          }
          frame "Basic" {
            n172 = call <vilib>:"WPI_DashboardUpdateNames.vi"("Controls on Tab"=w306) -> ()  [unwired: 11 in]
          }
          frame "Test" {
            w318 = -2 ("Active Item:Row Number")
            n173 = Index Array(array=w312, index=w311) -> (element=w313:T35)
            n174 = Unbundle(w313) -> ("Operation"=w314:enum16{"Update", "Clear"}, "Color Box"=w315:u32)
            n175 = call <vilib>:"NT Read and Format Entries as Tree.vi"("Operation"=w314, "Name Pattern"=w319, "Tree Refnum"=w320) -> ()  [unwired: 7 in, 2 out]
            n176 = call <vilib>:"NT Read String.vi"("Name"="TestMode/TestName") -> ("String"=w309:string)  [unwired: 9 in, 1 out]
            n177 = case shown="\"\"" w309 {
              tunnel: "TestMode/TestProgress" ("Name") -> [w322 _]
              tunnel: "TestMode/TestProgressText" ("Name") -> [w321 _]
              frame Default {
                n178 = call <vilib>:"NT Read Number.vi"("Name"=w322) -> ("Numeric"=w323:dbl)  [unwired: 9 in, 1 out]
                n179 = call <vilib>:"NT Read String.vi"("Name"=w321) -> ("String"=w324:string)  [unwired: 9 in, 1 out]
                n180 = Bundle("Numeric"=w323, "String"=w324) -> (→"Progress":cluster{"Numeric":dbl, "String":string})  [unwired: 1 in]
              }
              frame "" {
                n181 = local write "Test Name"(u16 0) -> ()
                n182 = property on="Progress" class="Clust (strict)"("Visible"=FALSE) -> ()  [unwired: 2 in, 2 out]
              }
            }
            n183 = property on="Test Tree" class="Tree (strict)"("Active Item Row Number"=w318, "ActiveColNum"=w318, "CellBG"=w315, "Active Item Row Number"=-1 ("Active Item:Row Number"), "CellBG"=u32 5789784 ("Color Box")) -> ()  [unwired: 2 in, 2 out]
          }
          frame "Variables" {
            w330 = string[] ["CameraPublisher", "Usage", "DB"]  # Items to initially close
            n184 = First Call?() -> (First Call?: T/F=w331:bool)
            n185 = control-ref of="Tree"() -> (w332:refnum<vi>)
            n186 = Select(t=w330, s=w331, f=string[] []) -> (s? t:f=w328:string[])
            n187 = call <vilib>:"NT Read and Format Entries as Tree.vi"("Tags to  Close"=w328, "Tree Refnum"=w332) -> ()  [unwired: 8 in, 2 out]
          }
          frame "Commands" {
            w341 = u32 5789784 ("Color Box")
            w342 = T36 {"Row"=-1, "Column"=-2} ("Active Cell:Active Cell")
            w344 = T36 {"Row"=-2, "Column"=-2} ("Active Cell:Active Cell")
            n188 = Index Array(array=w340, index=w339) -> (element=w338:T35)
            n189 = Index Array(array=w345, index=w339) -> (element=w343:u32)
            n190 = local read "Command Selection"() -> (w336:i32)
            n191 = property on="Command Params" class="Tbl (strict)"("Active Cell"=w344, "Cell BG Color"=w343, "Active Cell"=w342, "Cell BG Color"=w341) -> ()  [unwired: 2 in, 2 out]
            n192 = property on="Command Selection" class="MCListbox (strict)"("ActiveCell"=w344, "CellBG"=w343, "ActiveCell"=w342, "CellBG"=w341) -> ()  [unwired: 2 in, 2 out]
            n193 = Unbundle(w338) -> ("Operation"=w337:enum16{"Update", "Clear"})  [unwired: 1 out]
            n194 = call <vilib>:"WPI_DashboardUpdate RPC Info.vi"("Operation"=w337) -> ("update"=w335:bool, "commands"=w334:string[][])  [unwired: 9 in]
            n195 = property on="Command Selection" class="MCListbox (strict)"("ItemNames"=w334) -> ()  [unwired: 2 in, 2 out]
            n196 = call <vilib>:"WPI_DashboardUpdate Command Params.vi"("Update"=w335, "NewVal"=w336, "Commands"=w334, "Param Tbl"=w333) -> ()  [unwired: 7 in, 1 out]
          }
        }
      }
      event "Test Tree": Value Change {
        # "Show appropriate\ncontrols"
        n197 = event-data() -> ("CtlRef"=w350:refnum<vi>, "NewVal"=w348:string)  [unwired: 1 in]
        n198 = property on="Progress" class="Clust (strict)"("Visible"=FALSE) -> ()  [unwired: 2 in, 2 out]
        n199 = call <vilib>:"WPI_UtilitiesGetTreeIOName.vi"("NewVal"=w348, "TreeControl in"=w350) -> ("I/O Name"=w351:string)  [unwired: 9 in]
        n200 = case shown="\"Camera\"" w351 {
          selector: w351 -> [_ w358 _ w380 w389 _]
          tunnel: w348 -> [_ _ w377 w379 _ w396]
          tunnel: cluster{string[]}[] [{["640x480", "320x240", "160x120"]}, {["Auto", "Fixed indoor", "Fixed outdoor 1", "Fixed outdoor 2", "Fixed fluorescent 1", "Fixed fluorescent 2", "Hold current"]}, {["Auto", "Flicker-free 50 Hz", "Flicker-free 60 Hz", "Hold current"]}, {["None", "Prioritize frame rate", "Prioritize image quality"]}, {["Monochrome", "Color"]}] -> [_ _ _ _ _ w395]
          frame Default {
            w353 = FALSE ("Visible")
            w352 = FALSE ("Visible")
            n201 = property on="Test Slider" class="Slide (strict)"("Visible"=w353) -> ()  [unwired: 2 in, 2 out]
            n202 = property on="On/Off" class="Bool (strict)"("Visible"=w353) -> ()  [unwired: 2 in, 2 out]
            n203 = property on="Rev/Fwd" class="Clust (strict)"("Visible"=w353) -> ()  [unwired: 2 in, 2 out]
            n204 = property on="Test Ring" class="Ring (strict)"("Visible"=w352) -> ()  [unwired: 2 in, 2 out]
            n205 = property on="Motor" class="Clust (strict)"("Visible"=w352) -> ()  [unwired: 2 in, 2 out]
          }
          frame "Analog Out", "Motor", "PWM" {
            w359 = FALSE ("Visible")
            n206 = case shown="\"Analog Out\"" w358 {
              tunnel: [1.0 ("Value") -1.0 ("Value") 0.0 ("Value")] -> w357
              tunnel: [255.0 ("Value") 1.0 ("Value") 5.0 ("Value")] -> w356
              tunnel: [128.0 ("Value") 0.0 ("Value") 0.0 ("Value")] -> w355
              tunnel: [64.0 ("Value") 0.5 ("Value") 1.0 ("Value")] -> w354
              frame "PWM" {
              }
              frame "Motor", Default {
              }
              frame "Analog Out" {
              }
            }
            n207 = property on="Test Slider" class="Slide (strict)"("Visible"=w359) -> ()  [unwired: 2 in, 2 out]
            n208 = property on="Test Ring" class="Ring (strict)"("Visible"=w359) -> ()  [unwired: 2 in, 2 out]
            n209 = property on="On/Off" class="Bool (strict)"("Visible"=w359) -> ()  [unwired: 2 in, 2 out]
            n210 = property on="Rev/Fwd" class="Clust (strict)"("Visible"=w359) -> ()  [unwired: 2 in, 2 out]
            n211 = property on="Motor" class="Clust (strict)"("Visible"=TRUE) -> ()  [unwired: 2 in, 2 out]
            n212 = property on="Value" class="Slide (strict)"("Value"=w355, "Scale.Minimum"=w357, "Scale.Maximum"=w356, "Scale.Increment"=w354) -> ()  [unwired: 2 in, 2 out]
          }
          frame "Servo" {
            w375 = FALSE ("Visible")
            n213 = call <vilib>:"NT Read Number.vi"("Name"=w377) -> ("Numeric"=w376:dbl)  [unwired: 9 in, 1 out]
            n214 = property on="Test Slider" class="Slide (strict)"("Visible"=TRUE, "Scale.Maximum"=170.0 ("Scale.Range:Maximum")) -> ()  [unwired: 2 in, 2 out]
            n215 = local write "Test Slider"(w376) -> ()
            n216 = property on="Motor" class="Clust (strict)"("Visible"=w375) -> ()  [unwired: 2 in, 2 out]
            n217 = property on="Test Ring" class="Ring (strict)"("Visible"=w375) -> ()  [unwired: 2 in, 2 out]
            n218 = property on="On/Off" class="Bool (strict)"("Visible"=w375) -> ()  [unwired: 2 in, 2 out]
            n219 = property on="Rev/Fwd" class="Clust (strict)"("Visible"=w375) -> ()  [unwired: 2 in, 2 out]
          }
          frame "Relay", "Solenoid" {
            w378 = FALSE ("Visible")
            n220 = property on="Motor" class="Clust (strict)"("Visible"=w378) -> ()  [unwired: 2 in, 2 out]
            n221 = property on="Test Slider" class="Slide (strict)"("Visible"=w378) -> ()  [unwired: 2 in, 2 out]
            n222 = property on="Test Ring" class="Ring (strict)"("Visible"=w378) -> ()  [unwired: 2 in, 2 out]
            n223 = Search and Replace String(input string=w379, search string="/Value  **", replace string="/Direction") -> (result string=w385:string)  [unwired: 5 in, 3 out]
            n224 = call <vilib>:"NT Read String.vi"("Name"=w385) -> ("String"=w383:string)  [unwired: 9 in, 1 out]
            n225 = Equal?(x="Both directions", y=w383) -> (x = y?=w381:bool)
            n226 = property on="Rev/Fwd" class="Clust (strict)"("Visible"=w381) -> ()  [unwired: 2 in, 2 out]
            n227 = Not(x=w381) -> (.not. x?=w382:bool)
            n228 = property on="On/Off" class="Bool (strict)"("Visible"=w382, "Caption.Text"=w380) -> ()  [unwired: 2 in, 2 out]
          }
          frame "Compressor", "Digital Out" {
            w388 = FALSE ("Visible")
            # "Get direction and finish"
            n229 = property on="Test Ring" class="Ring (strict)"("Visible"=w388) -> ()  [unwired: 2 in, 2 out]
            n230 = property on="Motor" class="Clust (strict)"("Visible"=w388) -> ()  [unwired: 2 in, 2 out]
            n231 = property on="Test Slider" class="Slide (strict)"("Visible"=w388) -> ()  [unwired: 2 in, 2 out]
            n232 = property on="Rev/Fwd" class="Clust (strict)"("Visible"=FALSE) -> ()  [unwired: 2 in, 2 out]
            n233 = property on="On/Off" class="Bool (strict)"("Visible"=TRUE, "Caption.Text"=w389) -> ()  [unwired: 2 in, 2 out]
          }
          frame "Camera" {
            n234 = call <vilib>:"Get Last Path Segment.vi"("String in"=w396) -> ("String out"=w397:string)  [unwired: 10 in]
            n235 = property on="Motor" class="Clust (strict)"("Visible"=FALSE) -> ()  [unwired: 2 in, 2 out]
            n236 = property on="Rev/Fwd" class="Clust (strict)"("Visible"=FALSE) -> ()  [unwired: 2 in, 2 out]
            n237 = property on="On/Off" class="Bool (strict)"("Visible"=FALSE) -> ()  [unwired: 2 in, 2 out]
            n238 = case shown="\"White Balance  **\"" w397 {
              tunnel: w396 -> [w403 w412 w421 w430 w439 _ w445]
              tunnel: w395 -> [w401 w409 w418 w427 w436 _ _]
              frame "Size  **" {
                n239 = Index Array(array=w401) -> (element=w400:cluster{string[]})  [unwired: 1 in]
                n240 = call <vilib>:"NT Read String.vi"("Name"=w403) -> ("String"=w402:string)  [unwired: 9 in, 1 out]
                n241 = property on="Test Slider" class="Slide (strict)"("Visible"=FALSE) -> ()  [unwired: 2 in, 2 out]
                n242 = property on="Test Ring" class="Ring (strict)"("Visible"=TRUE) -> ()  [unwired: 2 in, 2 out]
                n243 = Unbundle(w400) -> (w398:string[])
                n244 = Match First String(2:w398, 3:w402) -> (0:w399:i32)  [unwired: 1 out]
                n245 = property on="Test Ring" class="Ring (strict)"("Value"=w399, "Strings []"=w398) -> ()  [unwired: 2 in, 2 out]
              }
              frame "White Balance  **" {
                n246 = call <vilib>:"NT Read String.vi"("Name"=w412) -> ("String"=w411:string)  [unwired: 9 in, 1 out]
                n247 = Index Array(array=w409, index=1) -> (element=w410:cluster{string[]})
                n248 = property on="Test Slider" class="Slide (strict)"("Visible"=FALSE) -> ()  [unwired: 2 in, 2 out]
                n249 = property on="Test Ring" class="Ring (strict)"("Visible"=TRUE) -> ()  [unwired: 2 in, 2 out]
                n250 = Unbundle(w410) -> (w407:string[])
                n251 = Match First String(2:w407, 3:w411) -> (0:w406:i32)  [unwired: 1 out]
                n252 = property on="Test Ring" class="Ring (strict)"("Value"=w406, "Strings []"=w407) -> ()  [unwired: 2 in, 2 out]
              }
              frame "Exposure  **" {
                n253 = call <vilib>:"NT Read String.vi"("Name"=w421) -> ("String"=w420:string)  [unwired: 9 in, 1 out]
                n254 = Index Array(array=w418, index=2) -> (element=w419:cluster{string[]})
                n255 = property on="Test Slider" class="Slide (strict)"("Visible"=FALSE) -> ()  [unwired: 2 in, 2 out]
                n256 = property on="Test Ring" class="Ring (strict)"("Visible"=TRUE) -> ()  [unwired: 2 in, 2 out]
                n257 = Unbundle(w419) -> (w415:string[])
                n258 = Match First String(2:w415, 3:w420) -> (0:w416:i32)  [unwired: 1 out]
                n259 = property on="Test Ring" class="Ring (strict)"("Value"=w416, "Strings []"=w415) -> ()  [unwired: 2 in, 2 out]
              }
              frame "Exposure Priority  **" {
                n260 = call <vilib>:"NT Read String.vi"("Name"=w430) -> ("String"=w429:string)  [unwired: 9 in, 1 out]
                n261 = Index Array(array=w427, index=3) -> (element=w428:cluster{string[]})
                n262 = property on="Test Slider" class="Slide (strict)"("Visible"=FALSE) -> ()  [unwired: 2 in, 2 out]
                n263 = property on="Test Ring" class="Ring (strict)"("Visible"=TRUE) -> ()  [unwired: 2 in, 2 out]
                n264 = Unbundle(w428) -> (w424:string[])
                n265 = Match First String(2:w424, 3:w429) -> (0:w425:i32)  [unwired: 1 out]
                n266 = property on="Test Ring" class="Ring (strict)"("Value"=w425, "Strings []"=w424) -> ()  [unwired: 2 in, 2 out]
              }
              frame "Color Enable  **" {
                n267 = call <vilib>:"NT Read String.vi"("Name"=w439) -> ("String"=w438:string)  [unwired: 9 in, 1 out]
                n268 = Index Array(array=w436, index=4) -> (element=w437:cluster{string[]})
                n269 = property on="Test Slider" class="Slide (strict)"("Visible"=FALSE) -> ()  [unwired: 2 in, 2 out]
                n270 = property on="Test Ring" class="Ring (strict)"("Visible"=TRUE) -> ()  [unwired: 2 in, 2 out]
                n271 = Unbundle(w437) -> (w433:string[])
                n272 = Match First String(2:w433, 3:w438) -> (0:w434:i32)  [unwired: 1 out]
                n273 = property on="Test Ring" class="Ring (strict)"("Value"=w434, "Strings []"=w433) -> ()  [unwired: 2 in, 2 out]
              }
              frame Default {
                n274 = property on="Test Slider" class="Slide (strict)"("Visible"=FALSE) -> ()  [unwired: 2 in, 2 out]
                n275 = property on="Test Ring" class="Ring (strict)"("Visible"=FALSE) -> ()  [unwired: 2 in, 2 out]
              }
              frame "Brightness  **", "Color Level  **", "Compression  **", "FPS  **", "Sharpness  **" {
                n276 = call <vilib>:"NT Read Number.vi"("Name"=w445) -> ("Numeric"=w444:dbl)  [unwired: 9 in, 1 out]
                n277 = property on="Test Slider" class="Slide (strict)"("Visible"=TRUE, "Scale.Maximum"=100.0 ("Scale.Range:Maximum")) -> ()  [unwired: 2 in, 2 out]
                n278 = local write "Test Slider"(w444) -> ()
                n279 = property on="Test Ring" class="Ring (strict)"("Visible"=FALSE) -> ()  [unwired: 2 in, 2 out]
              }
            }
          }
        }
      }
      event "Test Name": Mouse Enter {
        # "Populate the ring with the list of tests"
        n280 = event-data() -> ()  [unwired: 1 in, 1 out]
        n281 = call <vilib>:"NT Read String Array.vi"("Name"="TestMode/TestList") -> ("String Array"=w453:string[])  [unwired: 9 in, 1 out]
        n282 = Build Array (concatenate)("Select the test to run...", w453) -> (w452:string[])
        n283 = property on="Test Name" class="Ring (strict)"("Strings []"=w452) -> ()  [unwired: 2 in, 2 out]
      }
      event "Test Name": Value Change {
        w455 = FALSE ("Visible")
        # "Tell the robot the test name to run"
        n284 = event-data() -> ("NewVal"=w459:u16)  [unwired: 1 in]
        n285 = property on="Test Name" class="Ring (strict)"() -> ("Strings []"=w460:string[])  [unwired: 2 in, 2 out]
        n286 = local write "Progress"(T7 {"Test Progress"=0, "Test Progress Text"=""} ("Progress")) -> ()
        n287 = property on="Test Ring" class="Ring (strict)"("Visible"=w455) -> ()  [unwired: 2 in, 2 out]
        n288 = property on="Motor" class="Clust (strict)"("Visible"=w455) -> ()  [unwired: 2 in, 2 out]
        n289 = property on="Test Slider" class="Slide (strict)"("Visible"=w455) -> ()  [unwired: 2 in, 2 out]
        n290 = property on="On/Off" class="Bool (strict)"("Visible"=w455) -> ()  [unwired: 2 in, 2 out]
        n291 = property on="Rev/Fwd" class="Clust (strict)"("Visible"=w455) -> ()  [unwired: 2 in, 2 out]
        n292 = property on="Progress" class="Clust (strict)"("Visible"=TRUE) -> ()  [unwired: 2 in, 2 out]
        n293 = Index Array(array=w460, index=w459) -> (element=w458:string)
        n294 = call <vilib>:"NT Write String.vi"("String"=w458, "Name"="TestMode/TestName") -> ()  [unwired: 9 in, 1 out]
      }
      event "Select Auto": Mouse Enter {
        # "Populate the combo box with the list of autonomous options"
        n295 = event-data() -> ()  [unwired: 1 in, 1 out]
        n296 = call <vilib>:"NT Read String Array.vi"("Name"="Auto List") -> ("String Array"=w462:string[])  [unwired: 9 in, 1 out]
        n297 = property on="Select Auto" class="CmbBox"("Strings[]"=w462) -> ()  [unwired: 2 in, 2 out]
      }
      event "Select Auto": Value Change {
        # "User modified the Auto Selection. Write to NT variable so robot knows."
        n298 = event-data() -> ("NewVal"=w465:string)  [unwired: 1 in]
        n299 = call <vilib>:"NT Write String.vi"("String"=w465, "Name"="Auto Selector") -> ()  [unwired: 9 in, 1 out]
      }
      event "Command Selection": Value Change {
        # "Get the params and show in table"
        n300 = event-data() -> ("NewVal"=w471:i32)  [unwired: 1 in]
        n301 = property on="Command Selection" class="MCListbox (strict)"() -> ("ItemNames"=w469:string[][])  [unwired: 2 in, 2 out]
        n302 = call <vilib>:"WPI_DashboardUpdate Command Params.vi"("NewVal"=w471, "Commands"=w469, "Param Tbl"=w470) -> ()  [unwired: 8 in, 1 out]
      }
      event "Execute Command": Value Change {
        # "Started one, Unique ID holds\nresponse"
        n303 = event-data() -> ()  [unwired: 1 in, 1 out]
        n304 = property on="Command Selection" class="MCListbox (strict)"() -> ("ItemNames"=w482:string[][])  [unwired: 2 in, 2 out]
        n305 = Index Array(array=w482, index (row)="Command Selection", index (col)=0) -> (element=w480:string)
        n306 = call <vilib>:"Invoke Commands.vi"("Command Params"="Command Params", "Function Name"=w480) -> ("Params"=w476:u8, "Started"=w475:bool)  [unwired: 7 in, 1 out]
        n307 = Array Subset(array="Command Params", length (row)=w476) -> (w477:string[][])  [unwired: 3 in]
        n308 = Select(t="Executing" ("Cmd Status"), s=w475, f="" ("Cmd Status")) -> (s? t:f=→"Cmd Status":string)
      }
      event "Command Selection": Double Click {
        n309 = event-data() -> ("Row"=w490:i32)  [unwired: 1 in]
        n310 = property on="Command Selection" class="MCListbox (strict)"() -> ("ItemNames"=w493:string[][])  [unwired: 2 in, 2 out]
        n311 = local read "Command Params"() -> (w489:string[][])
        n312 = Index Array(array=w493, index (row)=w490, index (col)=0) -> (element=w491:string)
        n313 = call <vilib>:"Invoke Commands.vi"("Command Params"=w489, "Function Name"=w491) -> ("Params"=w488:u8, "Started"=w483:bool)  [unwired: 7 in, 1 out]
        n314 = Array Subset(array=w489, length (row)=w488) -> (w487:string[][])  [unwired: 3 in]
        n315 = Select(t="Executing" ("Cmd Status"), s=w483, f="" ("Cmd Status")) -> (s? t:f=w484:string)
        n316 = local write "Cmd Status"(w484) -> ()
      }
      event "CheckList": Double Click {
        # "Shift clears all"
        # "Update symbols on the listbox"
        n317 = event-data() -> ("PlatMods.Shift"=w495:bool, "Row"=w497:i32)  [unwired: 1 in]
        n318 = case shown="True" w495 {
          tunnel: w497 -> [w501 _]
          tunnel: 1 -> [w500 _]
          frame False {
            n319 = property on="CheckList" class="LstBox (strict)"() -> ("Item Symbols"=w499:i32[])  [unwired: 2 in, 2 out]
            n320 = Replace Array Subset(array=w499, new element=w500, index=w501) -> (w498:i32[])
            n321 = property on="CheckList" class="LstBox (strict)"("Item Symbols"=w498) -> ()  [unwired: 2 in, 2 out]
          }
          frame True {
            w502 = 0 ("Top Row")
            n322 = property on="CheckList" class="LstBox (strict)"() -> ("Number of Rows"=w504:u32)  [unwired: 2 in, 2 out]
            n323 = Initialize Array(0, w504) -> (w503:i32[])
            n324 = property on="CheckList" class="LstBox (strict)"("Top Row"=w502, "Value"=w502, "Item Symbols"=w503) -> ()  [unwired: 2 in, 2 out]
          }
        }
      }
      event "CheckList": Key Down {
        # "Update symbols on the listbox\nLeft and right keys check and uncheck"
        n325 = event-data() -> ("VKey"=w508:T33)  [unwired: 1 in]
        n326 = case shown="\"Left\", \"Right\"" w508 {
          selector: w508 -> [w513 _]
          tunnel: eventvkey."Left" ("VKey") -> [w511 _]
          frame "Left", "Right" {
            n327 = Equal?(x=w511, y=w513) -> (x = y?=w512:bool)
            n328 = Select(t=0, s=w512, f=1) -> (s? t:f=w514:i32)
            n329 = property on="CheckList" class="LstBox (strict)"() -> ("Item Symbols"=w517:i32[])  [unwired: 2 in, 2 out]
            n330 = Replace Array Subset(array=w517, new element=w514, index="CheckList") -> (w516:i32[])
            n331 = property on="CheckList" class="LstBox (strict)"("Item Symbols"=w516) -> ()  [unwired: 2 in, 2 out]
          }
          frame Default {
          }
        }
      }
      event "Motor.Enable": Value Change {
        # "When the test mode otor enable helper is set, update that\ntree row item's value"
        n332 = event-data() -> ("NewVal"=w523:bool)  [unwired: 1 in]
        n333 = Unbundle("Motor") -> ("Value"=w522:dbl)  [unwired: 1 out]
        n334 = Select(t=w522, s=w523, f=0.0) -> (s? t:f=w520:dbl)
        n335 = call <vilib>:"NT Write Number.vi"("Numeric"=w520, "Name"=w519) -> ()  [unwired: 9 in, 1 out]
      }
      event "Test Slider": Value Change {
        # "When the test mode slider helper is set, update that\ntree row item's value"
        n336 = event-data() -> ("NewVal"=w526:dbl)  [unwired: 1 in]
        n337 = call <vilib>:"NT Write Number.vi"("Numeric"=w526, "Name"=w527) -> ()  [unwired: 9 in, 1 out]
      }
      event "On/Off": Value Change {
        # "When the test mode on/off helper value is set, update that\ntree row item's value"
        n338 = event-data() -> ("NewVal"=w531:bool)  [unwired: 1 in]
        n339 = Boolean To (0,1)(Boolean=w531) -> (0, 1=w530:i16)
        n340 = call <vilib>:"NT Write Number.vi"("Numeric"=w530, "Name"=w529) -> ()  [unwired: 9 in, 1 out]
      }
      event "Rev/Fwd": Value Change {
        # "When the test mode helper value for relays is set, update that\ntree row item's value"
        n341 = event-data() -> ("NewVal.Forward"=w539:bool, "NewVal.Reverse"=w538:bool)  [unwired: 1 in]
        n342 = Boolean To (0,1)(Boolean=w539) -> (0, 1=w535:i16)
        n343 = Boolean To (0,1)(Boolean=w538) -> (0, 1=w537:i16)
        n344 = Negate(x=w537) -> (-x=w536:i16)
        n345 = Add(x=w535, y=w536) -> (x+y=w534:i16)
        n346 = call <vilib>:"NT Write Number.vi"("Numeric"=w534, "Name"=w533) -> ()  [unwired: 9 in, 1 out]
      }
      event "Test Ring": Value Change {
        # "When a test mode helper value is selected from the ring,\nset the tree item's variable to the string value"
        n347 = event-data() -> ("NewVal"=w543:u16)  [unwired: 1 in]
        n348 = property on="Test Ring" class="Ring (strict)"() -> ("Strings []"=w544:string[])  [unwired: 2 in, 2 out]
        n349 = Index Array(array=w544, index=w543) -> (element=w542:string)
        n350 = call <vilib>:"NT Write String.vi"("String"=w542, "Name"=w541) -> ()  [unwired: 9 in, 1 out]
      }
      event "Rec Mode": Value Change {
        # "Update globals for recording mode and path to read log from.\nClear when logging and let NetworkTables set path for vision to\nuse."
        n351 = event-data() -> ("NewVal"=w555:enum32{"Stop", "Record", "Playback"})  [unwired: 1 in]
        n352 = global write "WPI_DashboardLogging Global.vi" "Logging Filename"(path "") -> ()
        n353 = global write "WPI_DashboardLogging Global.vi" "Recording"(w555) -> ()
        n354 = case shown="\"Playback\"" w555 {
          tunnel: w554 -> [_ w557 w566]
          tunnel: [_ _ w565] -> w552
          tunnel: [_ _ w564] -> _
          tunnel: w550 -> [_ _ w562]
          tunnel: cluster{i32, i32} {-250, 170} -> [_ _ w561]
          tunnel: [_ _ T34 {"Image Size"=TRUE, "Image Type"=TRUE, "Pixel Value"=TRUE, "ROI Information"=TRUE, "Zoom Factor"=FALSE} ("Image Information Shown:All Elements")] -> w545
          tunnel: [_ _ TRUE ("Zoom Factor")] -> w546
          tunnel: w548 -> [_ _ w558]
          frame Default {
          }
          frame "Stop", "Record" {
            # "Place Window too"
            n355 = invoke class="VI" method="FP.Close"(reference=w557) -> (reference out=w556:refnum<vi>)  [unwired: 2 in, 2 out]
            n356 = invoke class="VI" method="Abort VI"(reference=w556) -> ()  [unwired: 2 in, 3 out]
          }
          frame "Playback" {
            n357 = call "Open Playback Panel.vi"("Offset"=w561, "DB VI Ref"=w562, "Playback in"=w566) -> ("Playback out"=w563:refnum<vi>)  [unwired: 8 in]
            n358 = register-events(w563, w558) -> (reference out=w565:refnum<event-registration>, error out=w564:errorcluster)  [unwired: 2 in]
          }
        }
        n359 = property on="Camera Image" class="ImageControl"("Image Information Shown"=w545, "Image Information Visible"=w546) -> ()  [unwired: 2 in, 2 out]
        n360 = property on="Camera Image Right" class="ImageControl"("Image Information Shown"=w545, "Image Information Visible"=w546) -> ()  [unwired: 2 in, 2 out]
        n361 = call <vilib>:"WPI_DashboardNT Log FieldName Cache.vi"("Operation"=enum16{"Lookup/Add", "Index", "Clear"}."Clear") -> ()  [unwired: 8 in, 3 out]
      }
      event Panel Close {
        w568 = enum32{"Stop", "Record", "Playback"}."Stop" ("Rec Mode")
        # "Playback window has been closed, abort"
        n362 = event-data() -> ()  [unwired: 1 in, 4 out]
        n363 = local write "Rec Mode"(w568) -> ()
        n364 = global write "WPI_DashboardLogging Global.vi" "Recording"(w568) -> ()
      }
      event Panel Close {
        # "Abort playback window and ourself"
        n365 = event-data() -> ()  [unwired: 1 in, 4 out]
        n366 = invoke class="VI" method="FP.Close"(reference=w572) -> (reference out=w571:refnum<vi>)  [unwired: 2 in, 2 out]
        n367 = invoke class="VI" method="Abort VI"(reference=w571) -> (error out=w570:errorcluster)  [unwired: 2 in, 2 out]
        n368 = invoke class="VI" method="Abort VI"(error in=w570) -> ()  [unwired: 2 in, 3 out]
      }
      event User Event {
        n369 = event-data() -> ("IDs"=w579:cluster{"RPC field ID":u16, "Unique ID":u16}, "String"=w578:string)  [unwired: 1 in]
        n370 = local write "Cmd Status"("" ("Cmd Status")) -> ()
        n371 = Bundle("IDs"=w579, "String"=w578) -> (w577:T10)  [unwired: 1 in]
        n372 = call <vilib>:"Retrieve RPC Response.vi"("RPC Response"=w577) -> ("Output"=w575:string[][])  [unwired: 10 in]
        n373 = Build Array (concatenate)(w573, w575) -> (w574:string[][])
        n374 = local write "Command Params"(w574) -> ()
      }
      event "Tree": Double Click {
        n375 = event-data() -> ("PlatMods"=w585:T37, "Tag"=w582:string)  [unwired: 1 in]
        n376 = Unbundle(w585) -> ("Shift"=w584:bool)  [unwired: 4 out]
        n377 = Not(x=w584) -> (.not. x?=w583:bool)
        n378 = String Subset(string=w582, length (rest)=1 ("length (rest)")) -> (substring=w581:string)  [unwired: 1 in]
        n379 = case shown="\"/\"" w581 {
          tunnel: w582 -> [_ w588]
          tunnel: w583 -> [_ w587]
          frame Default {
          }
          frame "/" {
            n380 = call <vilib>:"NT Update Persistence.vi"("Persistence"=w587, "Name"=w588) -> ()  [unwired: 9 in, 1 out]
          }
        }
      }
    }
  }
  n381 = while {
    tunnel: w56 -> [w600]
    tunnel: w1 -> [w598]
    tunnel: [w596] -> _
    tunnel: u32 1000 ("milliseconds to wait") -> [w595]
    tunnel: w27 -> [w589]
    i -> [w596]
    stop <- FALSE stop-if-true
    n382 = Wait on Notification(notifier=w598, timeout in ms (-1)=w595) -> (notification=w597:string, timed out?=w593:bool)  [unwired: 2 in, 2 out]
    n383 = local read "Rec Mode"() -> (w591:enum32{"Stop", "Record", "Playback"})
    n384 = Equal?(x=w591, y=u16 2 ("Rec Mode")) -> (x = y?=w592:bool)
    n385 = Compound Arithmetic op=OR(invert w593, w592) -> (w594:bool)
    n386 = case shown="True" w594 {
      tunnel: w600 -> [_ w603]
      tunnel: w597 -> [_ w602]
      tunnel: w589 -> [_ w601]
      frame False {
      }
      frame True {
        n387 = call <vilib>:"Bind Controls to SmartDashboard.vi"("RPC ref"=w601, "Bound Control Refs"=w603, "Server IP Address"=w602) -> ()  [unwired: 9 in]
      }
    }
  }
